vi "000 Write TXT.vi"(8 "error in (no error)":errorcluster caption="Error In", 10 "txt":string, 11 "Path":path) -> (0 "error out":errorcluster caption="Error Out")   [LabVIEW 2020]
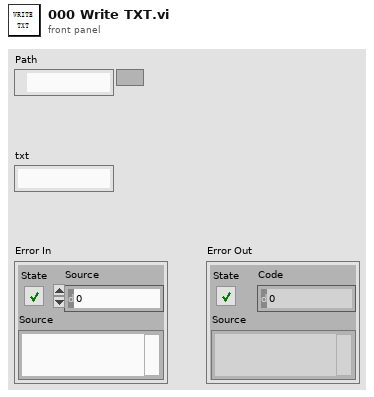
[diagram p1: front panel]
types:
  T1 = enum16{"open", "replace", "create", "open or create", "replace or create", "replace or create with confirmation"}
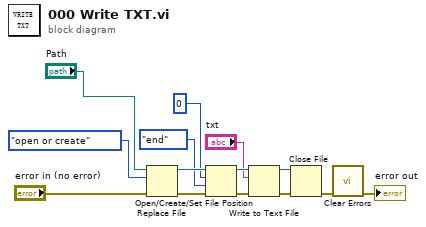
[diagram p0: block diagram]
diagram:
  n1 = Open/Create/Replace File(file path (use dialog)="Path", error in="error in (no error)", operation (0:open)=T1."open or create" ("操作(0:open)")) -> (refnum out=w11:refnum<file>, error out=w10:errorcluster)  [unwired: 3 in, 1 out]
  n2 = Set File Position(offset (in bytes) (0)=i64 0 ("偏移量（字节）（0）"), refnum=w11, from (0:start)=enum16{"start", "end", "current"}."end" ("自（0:起始）"), error in=w10) -> (refnum out=w9:refnum<file>, error out=w8:errorcluster)
  n3 = Write to Text File(file (use dialog)=w9, text="txt", error in=w8) -> (refnum out=w13:refnum<file>, error out=w14:errorcluster)  [unwired: 1 in, 1 out]
  n4 = Close File(refnum=w13, error in=w14) -> (error out=w5:errorcluster)  [unwired: 1 out]
  n5 = call <vilib>:"Clear Errors.vi"("error in (no error)"=w5) -> ("error out"=→"error out":errorcluster)  [unwired: 5 in, 1 out]
